vi "Set ID.vi"(8 "error in (no error)":errorcluster, 10 "ID":i64, 11 "Challenge in":refnum<class "Challenge.lvclass">) -> (0 "error out":errorcluster, 3 "Challenge out":refnum<class "Challenge.lvclass">)   [LabVIEW 2020, in "Summer of LabVIEW.lvlib" / "Challenge.lvclass"]
uses:
  Challenge.lvclass
  Challenge.lvclass/Challenge.ctl
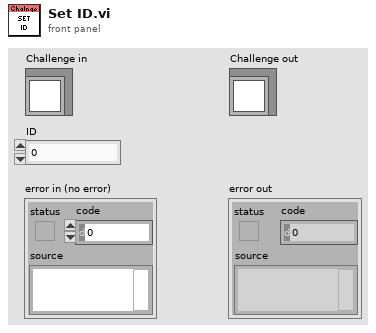
[diagram p1: front panel]
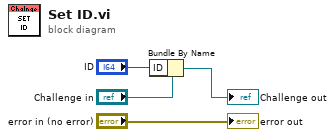
[diagram p0: block diagram]
diagram:
  n1 = Bundle By Name(cluster="Challenge in", "ID"="ID") -> (→"Challenge out":refnum<class "Challenge.lvclass">)
  "error out" <- "error in (no error)"
